vi "Start Measurement.vi"(8 "error in (no error)":errorcluster, 10 "Measurement Parameters":T1={"Start Step"=0, "End Step"=768, "Cluster Count"=1, "Scan Interval"=0, "Number of Scans"=0, "Measurement Type"=enum."MS"}, 11 "VISA Refnum in":refnum<visa-resource-name>) -> (0 "error out":errorcluster, 3 "VISA Refnum out":refnum<visa-resource-name>)   [LabVIEW 2016]
uses:
  Type Definitions/Controls/Measurement Parameters.ctl
  Type Definitions/Controls/Measurement Type.ctl
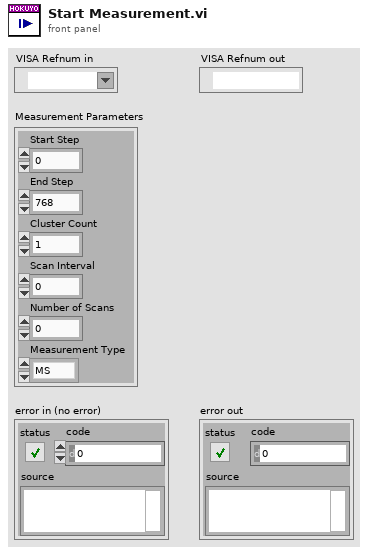
[diagram p1: front panel]
types:
  T1 = typedef "Measurement Parameters.ctl" = cluster{"Start Step":u32, "End Step":u32, "Cluster Count":u32, "Scan Interval":u32, "Number of Scans":u32, "Measurement Type":T2}
  T2 = typedef "Measurement Type.ctl" = enum16{"MS"}
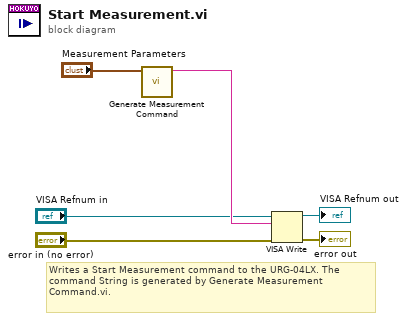
[diagram p0: block diagram]
diagram:
  # "Writes a Start Measurement command to the URG-04LX. The \ncommand String is generated by Generate Measurement Command.vi."
  n1 = call "Generate Measurement Command.vi"("Measurement Parameters"="Measurement Parameters") -> ("Measurement Command"=w5:string)  [unwired: 10 in]
  n2 = VISA Write(VISA resource name="VISA Refnum in", write buffer=w5, error in (no error)="error in (no error)") -> (VISA resource name out=→"VISA Refnum out":refnum<visa-resource-name>, error out=→"error out":errorcluster)  [unwired: 1 out]
